vi "Write enable.vi"(8 "error in (no error)":errorcluster, 10 "enable":bool, 11 "Enable Heater v MSG in":refnum<class "Enable Heater MSG.lvclass">) -> (0 "error out":errorcluster, 3 "Enable Heater v MSG out":refnum<class "Enable Heater MSG.lvclass">)   [LabVIEW 2017, in "Controller.lvlib" / "Enable Heater MSG.lvclass"]
uses:
  Enable Heater MSG.lvclass
  Enable Heater MSG.lvclass/Enable Heater MSG.ctl
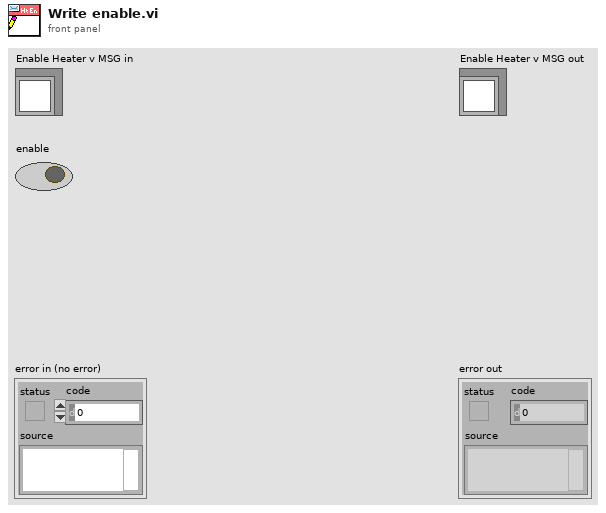
[diagram p1: front panel]
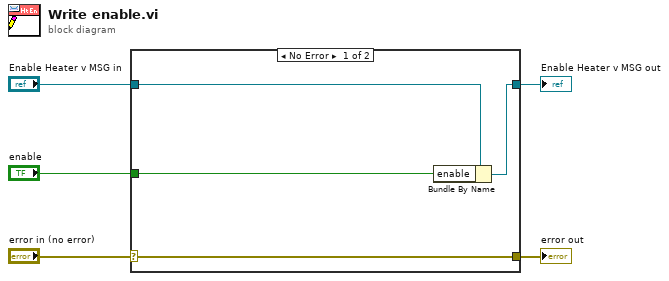
[diagram p0: block diagram]
diagram:
  n1 = case shown="No Error" "error in (no error)" {
    selector: "error in (no error)" -> [w9 w10]
    tunnel: [w9 w10] -> w4
    tunnel: [w7 w11] -> w2
    tunnel: "Enable Heater v MSG in" -> [w8 w11]
    tunnel: "enable" -> [w6 _]
    frame No Error {
      n2 = Bundle By Name(cluster=w8, "enable"=w6) -> (w7:refnum<class "Enable Heater MSG.lvclass">)
    }
    frame Error {
    }
  }
  "error out" <- w4
  "Enable Heater v MSG out" <- w2
